vi "LVClass_CorrectionDataManager GetInteractionMatrixData.vi"(0 "CorrectionDataManager in":refnum<class "CorrectionDataManager.lvclass">, 11 "error in (no error)":errorcluster) -> (4 "CorrectionDataManager out":refnum<class "CorrectionDataManager.lvclass">, 6 "Interaction matrix":sgl[][](array[numeric]), 15 "error out":errorcluster)   [LabVIEW 2020, in "CorrectionDataManager.lvclass"]
doc: "Interaction matrix content getter.\n\n<B>corrdata_managerIn</B> : CorrDataManager object.\n<B>corrdata_managerOut</B> : CorrDataManager object.\n<B>data</B> : 2D Array of interaction matrix content."
uses:
  CorrectionDataManager.lvclass
  CorrectionDataManager.lvclass/CorrectionDataManager.ctl
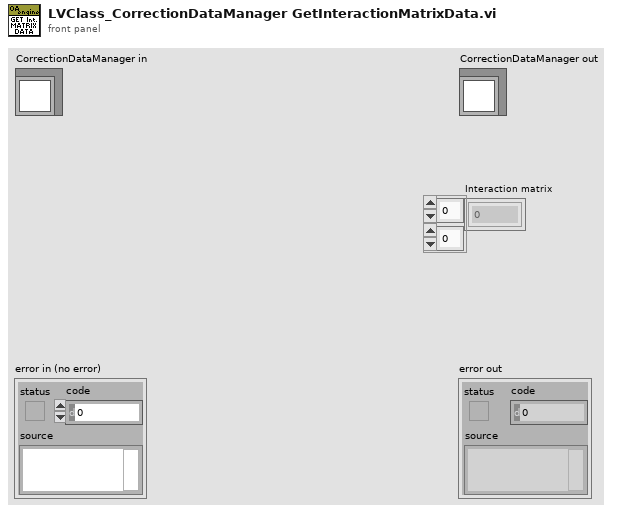
[diagram p1: front panel]
types:
  T1 = typedef "ClassID.ctl" = i64
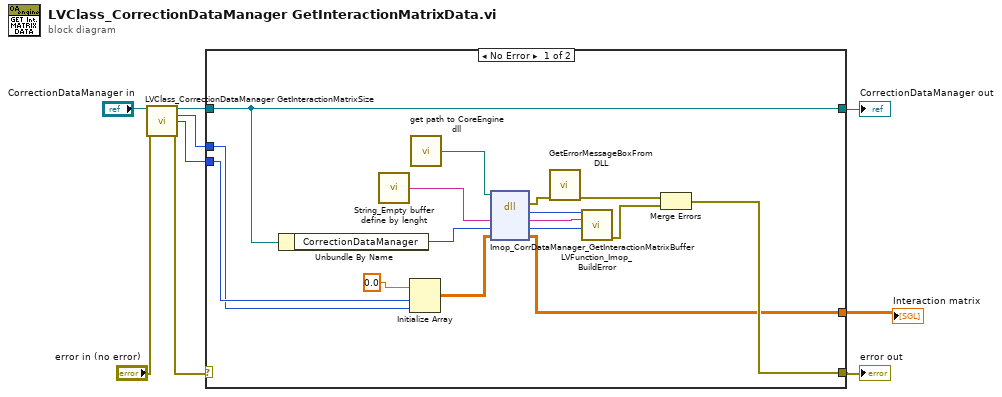
[diagram p0: block diagram]
diagram:
  n1 = call "LVClass_CorrectionDataManager GetInteractionMatrixSize.vi"("CorrectionDataManager in"="CorrectionDataManager in", "error in (no error)"="error in (no error)") -> ("CorrectionDataManager out"=w4:refnum<class "CorrectionDataManager.lvclass">, "# of valid actuators (nb col)"=w1:u32, "2 time of valid sub pupil (nb line)"=w3:u32, "error out"=w6:errorcluster)  [unwired: 10 in]
  n2 = case shown="No Error" w6 {
    selector: w6 -> [_ w27]
    tunnel: [w18 w27] -> w8
    tunnel: [w15 w26] -> w9
    tunnel: w4 -> [w15 w26]
    tunnel: w3 -> [w12 _]
    tunnel: [w13 _] -> w2
    tunnel: w1 -> [w11 _]
    frame No Error {
      n3 = Unbundle By Name(w15) -> ("CorrectionDataManager"=w17:T1)
      n4 = call "String_Empty buffer define by lenght.vi"() -> ("Empty buffer"=w23:string)  [unwired: 1 in]
      n5 = Initialize Array(sgl 0.0 ("Numeric"), w12, w11) -> (w14:sgl[][])
      n6 = call "get path to CoreEngine dll.vi"() -> ("path to wavekit library"=w22:path)  [unwired: 14 in, 1 out]
      n7 = dll-call lib="D:/soft/HASO_v3/SVN_trunk/ImOpCoreEngine4_LV2011/DLLs/c_interface_vc100.dll" fn="Imop_CorrDataManager_GetInteractionMatrixBuffer"(path in=w22, "message"=w23, "WavefrontCorrection"=w17, "Data Matrix"=w14) -> (error out=w21:errorcluster, "return type"=w25:i32, "message"=w24:string, "WavefrontCorrection"=w10:i64, "Data Matrix"=w13:sgl[][])  [unwired: 2 in, 1 out]
      n8 = call "GetErrorMessageBoxFromDLL.vi"("error IN"=w21) -> ("error OUT"=w20:errorcluster)  [unwired: 10 in]
      n9 = call "LVFunction_Imop_BuildError.vi"("code"=w25, "String to Prepend to source (\"\")"=w24, "Adresse"=w10) -> ("error out"=w19:errorcluster)  [unwired: 12 in]
      n10 = Merge Errors(w20, w19) -> (w18:errorcluster)
    }
    frame Error {
    }
  }
  "error out" <- w8
  "CorrectionDataManager out" <- w9
  "Interaction matrix" <- w2
